vi "macro_Angle_Modulus.vi"   [LabVIEW 2019, in "Trajectory_Library.lvlib"]
uses:
  Trajectory_Library.lvlib
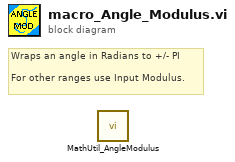
[diagram p0: block diagram]
diagram:
  # "Wraps an angle in Radians to +/- PI\n\nFor other ranges use Input Modulus."
  n1 = call "MathUtil_AngleModulus.vi"() -> ()  [unwired: 11 in, 1 out]
